vi "StopStreaming.vi"(8 "error in (no error)":errorcluster, 11 "Camera in":refnum<class "CameraI2COUSB.lvclass">) -> (0 "error out":errorcluster, 3 "Camera out":refnum<class "CameraI2COUSB.lvclass">)   [LabVIEW 2020, in "CameraI2COUSB.lvlib" / "CameraI2COUSB.lvclass"]
doc: "Stop streaming"
uses:
  CameraI2COUSB.lvclass
  CameraI2COUSB.lvclass/CameraI2COUSB.ctl
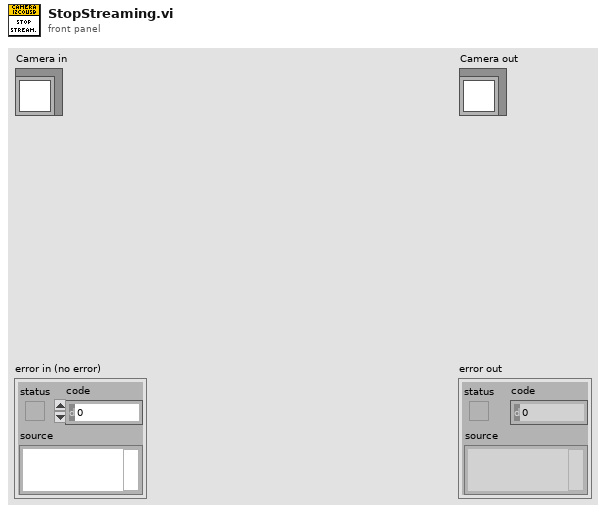
[diagram p1: front panel]
types:
  T1 = typedef "CameraI2COUSB.lvlib/CameraI2COUSB.lvclass/StopStreamingEvnt.ctl" = refnum<user-event>
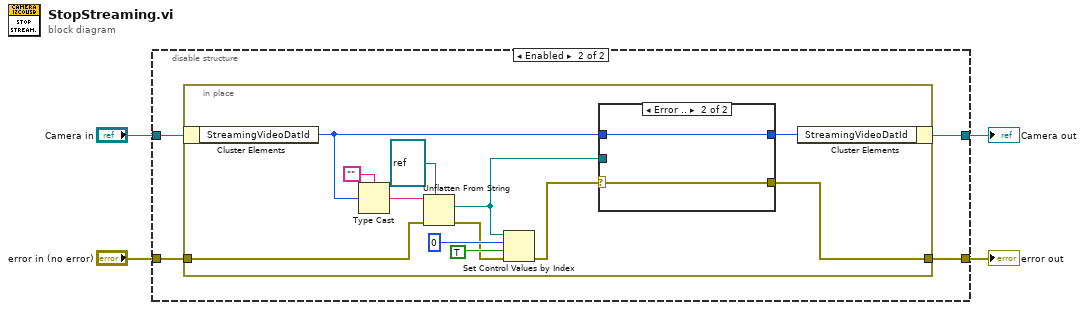
[diagram p0: block diagram]
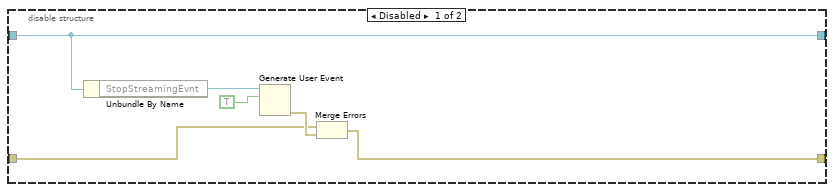
[diagram p2: hidden frame]
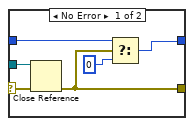
[diagram p3: hidden frame]
diagram:
  n1 = disable-structure shown="Enabled" {
    disable-tunnel: "Camera in" -> [w5 w12]
    disable-tunnel: [w7 w14] -> w3
    disable-tunnel: "error in (no error)" -> [w6 w13]
    disable-tunnel: [w5 w11] -> w1
    frame Disabled {
      n2 = Unbundle By Name(w5) -> ("StopStreamingEvnt"=w10:T1)
      n3 = Generate User Event(user event=w10, event data cluster=TRUE ("event data")) -> (error out=w8:errorcluster)  [unwired: 2 in, 1 out]
      n4 = Merge Errors(w6, w8) -> (w7:errorcluster)
    }
    frame Enabled {
      n5 = in-place {
        in-place-border: [w15] -> w14
        in-place-border: w13 -> [w22]
        n6 = in-place-cluster #1(w12) -> ("StreamingVideoDatId"=w17:u32)
        n7 = Type Cast(type="", x=w17) -> (*(type *) &x=w23:string)
        n8 = Unflatten From String(type=refnum<vi> refnum ("type specifier VI Refnum (for type only)"), binary string=w23, error in (no error)=w22) -> (value=w18:refnum<vi>, error out=w21:errorcluster)  [unwired: 2 in, 1 out]
        n9 = Set Control Values by Index(0:w18, 1:0, 2:TRUE, 3:w21) -> (11:w19:errorcluster)
        n10 = case shown="Error .." w19 {
          selector: w19 -> [w32 w34]
          tunnel: w18 -> [w31 _]
          tunnel: w17 -> [w30 w33]
          tunnel: [w28 w33] -> w16
          tunnel: [w27 w34] -> w15
          frame No Error {
            n11 = Close Reference(reference=w31, error in (no error)=w32) -> (error out=w27:errorcluster)
            n12 = Select(t=w30, s=w27, f=u32 0) -> (s? t:f=w28:u32)
          }
          frame Error {
          }
        }
        n13 = in-place-cluster #1("StreamingVideoDatId"=w16) -> (w11:refnum<class "CameraI2COUSB.lvclass">)
      }
    }
  }
  "error out" <- w3
  "Camera out" <- w1
